vi "Display Multiple Channels.vi"(8 "Error In":errorcluster, 10 "Single Channel?":bool, 11 "Waveform Array":waveform(dbl)[][](array[waveform])) -> (0 "Error Out":errorcluster, 1 "Trigger":dynamicdata(graph), 2 "Dev2 Ch3":dynamicdata(graph), 3 "Dev1 Ch3":dynamicdata(graph))   [LabVIEW 2017]
panel:
  out "Dev1":waveform(dbl)[](array[waveform])
  out "Dev2":waveform(dbl)[](array[waveform])
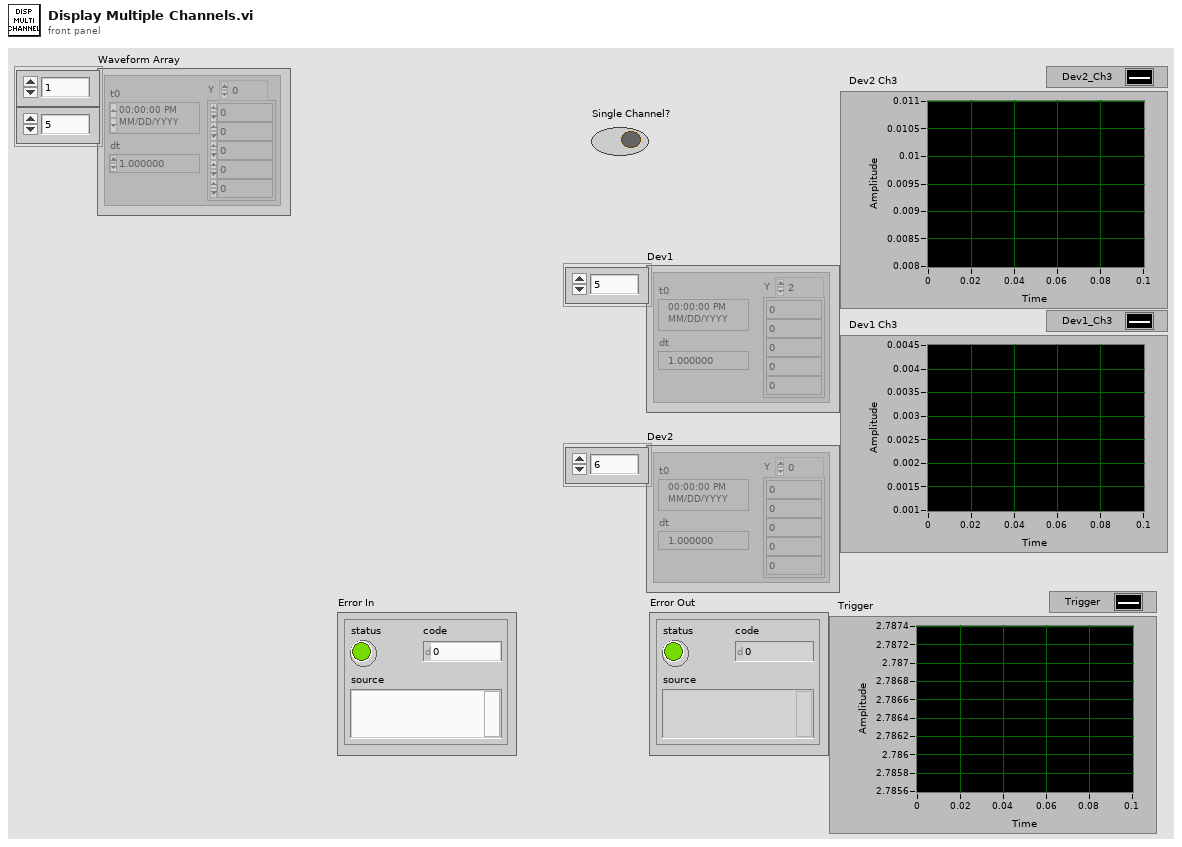
[diagram p1: front panel]
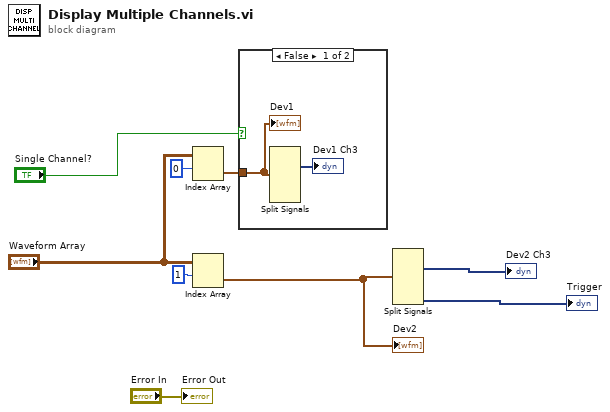
[diagram p0: block diagram]
diagram:
  n1 = Index Array(array="Waveform Array", index (row)=0) -> (element=w2:waveform(dbl)[])  [unwired: 1 in]
  n2 = Index Array(array="Waveform Array", index (row)=1) -> (element=w6:waveform(dbl)[])  [unwired: 1 in]
  "Dev2" <- w6
  n3 = case shown="False" "Single Channel?" {
    tunnel: w2 -> [w10 _]
    frame False {
      n4 = Split Signals(w10) -> (→"Dev1 Ch3":dynamicdata)  [unwired: 7 in, 6 out]
      "Dev1" <- w10
    }
    frame True {
    }
  }
  n5 = Split Signals(w6) -> (→"Dev2 Ch3":dynamicdata, →"Trigger":dynamicdata)  [unwired: 7 in, 5 out]
  "Error Out" <- "Error In"
